vi "Get Subsystem by Name.vi"(8 "error in (no error)":errorcluster, 10 "Name":string) -> (0 "error out":errorcluster, 1 "found":bool, 2 "Subsystem":refnum<class "SMO.lvclass">)   [LabVIEW 2013, in "Registry-SMO.lvclass"]
uses:
  Registry-SMO.lvclass
  SMO/SMO.lvclass
  Registry-SMO.lvclass/Registry-SMO.ctl
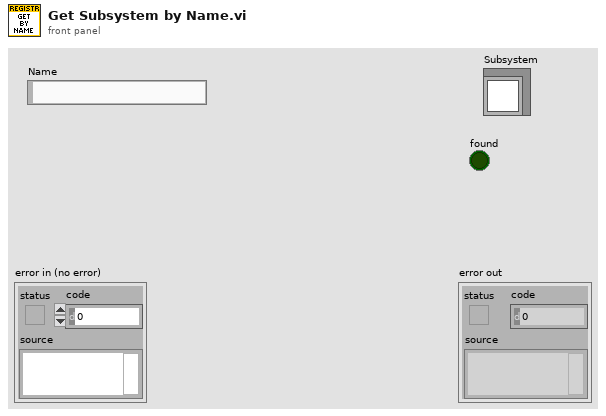
[diagram p1: front panel]
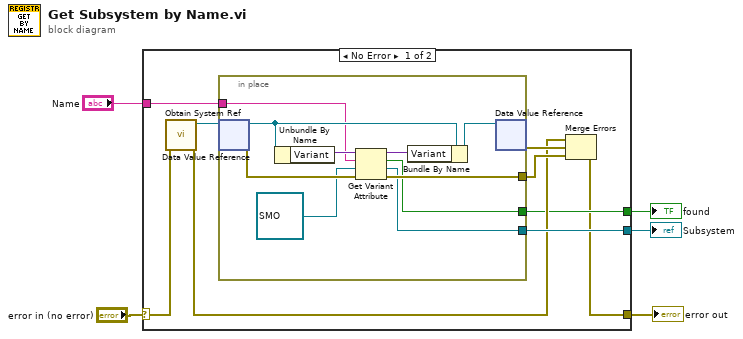
[diagram p0: block diagram]
diagram:
  n1 = case shown="No Error" "error in (no error)" {
    selector: "error in (no error)" -> [w10 w25]
    tunnel: [w6 w25] -> w4
    tunnel: [w12 _] -> w3
    tunnel: "Name" -> [w8 _]
    tunnel: [w7 _] -> w1
    frame No Error {
      n2 = call "Obtain System Ref.vi"("error in (no error)"=w10) -> ("error out"=w9:errorcluster, "JKI SMO System"=w11:refnum<data-value>)  [unwired: 9 in]
      n3 = in-place {
        in-place-border: [w19] -> w13
        in-place-border: [w16] -> w12
        in-place-border: w8 -> [w18]
        in-place-border: [w15] -> w7
        n4 = in-place-dvr #1(w11) -> (w24:refnum<class "Registry-SMO.lvclass">, w20:errorcluster)
        n5 = Unbundle By Name(w24) -> ("Variant"=w22:variant)
        n6 = Get Variant Attribute(Variant=w22, name=w18, default value (empty Variant)=refnum<class "SMO.lvclass"> refnum ("JKI SMO.lvclass"), error in=w20) -> (duplicate Variant=w21:variant, found=w15:bool, value=w16:refnum<class "SMO.lvclass">, error out=w19:errorcluster)
        n7 = Bundle By Name(cluster=w24, "Variant"=w21) -> (w23:refnum<class "Registry-SMO.lvclass">)
        n8 = in-place-dvr #1(w23) -> (w14:errorcluster)  [unwired: 1 out]
      }
      n9 = Merge Errors(w9, w14, w13) -> (w6:errorcluster)
    }
    frame Error {
    }
  }
  "error out" <- w4
  "Subsystem" <- w3
  "found" <- w1
